vi "CreateTimers.vi"() -> (4 "TimerRegisters":T1={"Tick0"="Tick0", "Tock0"="Tock0", "Tick1"="Tick1", "Tock1"="Tock1", "Tick2"="Tick1", "Tock2"="Tock1", "Tick3"="Tick1", "Tock3"="Tock1", "Tick4"="Tick0", "Tock4"="Tock0", "Tick5"="Tick1", "Tock5"="Tock1", "Tick6"="Tick1", "Tock6"="Tock1", "Tick7"="Tick1", "Tock7"="Tock1"})   [LabVIEW 2015, in "Timers.lvlib"]
doc: "Creates 16 registers (x8 Ticks and x8 Tocks) when in total allows 8 individual timers."
uses:
  Timers.lvlib
  TimerRegisters.ctl
  <vilib>/rvi/DataTransferAndStorage/Container/Common/niFpgaContainerGetUniqueNameForEmu.vi
  <vilib>/rvi/DataTransferAndStorage/Container/Common/niFpgaContainerSetEmuInfo.vi
  <vilib>/rvi/eio/common/nirviEmuReportErrorAndStop.vi
  <vilib>/rvi/LocalResourceManager/LocalResourceManager.xnode
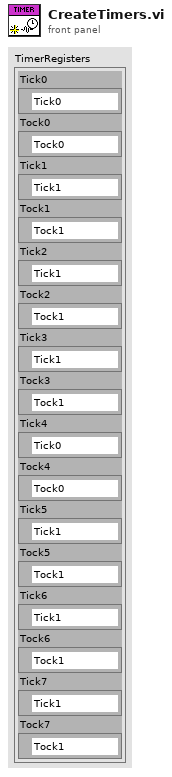
[diagram p1: front panel]
types:
  T1 = typedef "Timers.lvlib/TimerRegisters.ctl" = cluster{"Tick0":refnum<k21>, "Tock0":refnum<k21>, "Tick1":refnum<k21>, "Tock1":refnum<k21>, "Tick2":refnum<k21>, "Tock2":refnum<k21>, "Tick3":refnum<k21>, "Tock3":refnum<k21>, "Tick4":refnum<k21>, "Tock4":refnum<k21>, "Tick5":refnum<k21>, "Tock5":refnum<k21>, "Tick6":refnum<k21>, "Tock6":refnum<k21>, "Tick7":refnum<k21>, "Tock7":refnum<k21>}
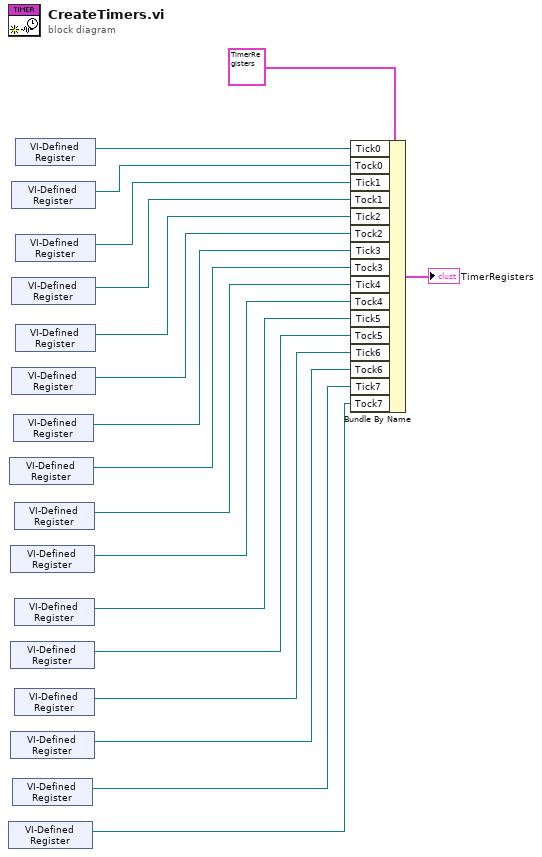
[diagram p0: block diagram]
diagram:
  n1 = xnode "VI-Defined Register"() -> ("Register Out"=w1:refnum<k21>)
  n2 = xnode "VI-Defined Register"() -> ("Register Out"=w9:refnum<k21>)
  n3 = xnode "VI-Defined Register"() -> ("Register Out"=w7:refnum<k21>)
  n4 = xnode "VI-Defined Register"() -> ("Register Out"=w5:refnum<k21>)
  n5 = xnode "VI-Defined Register"() -> ("Register Out"=w3:refnum<k21>)
  n6 = xnode "VI-Defined Register"() -> ("Register Out"=w16:refnum<k21>)
  n7 = xnode "VI-Defined Register"() -> ("Register Out"=w13:refnum<k21>)
  n8 = xnode "VI-Defined Register"() -> ("Register Out"=w11:refnum<k21>)
  n9 = xnode "VI-Defined Register"() -> ("Register Out"=w2:refnum<k21>)
  n10 = xnode "VI-Defined Register"() -> ("Register Out"=w10:refnum<k21>)
  n11 = xnode "VI-Defined Register"() -> ("Register Out"=w8:refnum<k21>)
  n12 = xnode "VI-Defined Register"() -> ("Register Out"=w6:refnum<k21>)
  n13 = xnode "VI-Defined Register"() -> ("Register Out"=w4:refnum<k21>)
  n14 = xnode "VI-Defined Register"() -> ("Register Out"=w17:refnum<k21>)
  n15 = xnode "VI-Defined Register"() -> ("Register Out"=w14:refnum<k21>)
  n16 = xnode "VI-Defined Register"() -> ("Register Out"=w12:refnum<k21>)
  n17 = Bundle By Name(cluster=T1 {"Tick0"="Tick0", "Tock0"="Tock0", "Tick1"="Tick1", "Tock1"="Tock1", "Tick2"="Tick1", "Tock2"="Tock1", "Tick3"="Tick1", "Tock3"="Tock1", "Tick4"="Tick0", "Tock4"="Tock0", "Tick5"="Tick1", "Tock5"="Tock1", "Tick6"="Tick1", "Tock6"="Tock1", "Tick7"="Tick1", "Tock7"="Tock1"} ("TimerRegisters"), "Tick0"=w17, "Tock0"=w16, "Tick1"=w14, "Tock1"=w13, "Tick2"=w12, "Tock2"=w11, "Tick3"=w10, "Tock3"=w9, "Tick4"=w8, "Tock4"=w7, "Tick5"=w6, "Tock5"=w5, "Tick6"=w4, "Tock6"=w3, "Tick7"=w2, "Tock7"=w1) -> (→"TimerRegisters":T1)
